vi "Configure Spot Frequency.vi"(0 "VISA resource name":refnum<visa-resource-name>, 1 "Spot Frequency Measurement Type (1: Signal Phase Noise)":i32(ring)=1 items=["Displayed Average Noise Level Floor", "Signal Phase Noise"], 2 "Video Resolution Bandwidth Ratio (1)":dbl=1.0, 3 "Average Count (0)":dbl, 4 "Averaging Method (0: Exponential)":i32(ring) items=["Exponential", "Repeat"], 5 "error in (no error)":errorcluster, 6 "Auto Phase Noise Optimization (T: Enable)":bool=TRUE, 7 "Spot Frequency Offset (10000 Hz)":dbl=10000.0 format="%^#_6g", 8 "Manual Phase Noise Optimization (45000 Hz)":dbl=45000.0 format="%^#_6g", 9 "Resolution Bandwidth (10%)":dbl=10.0, 11 "Sweep Time (0.005 s)":dbl=0.005) -> (14 "VISA resource name out":refnum<visa-resource-name>, 19 "error out":errorcluster)   [LabVIEW 2014, in "Agilent ESA PSA Series.lvlib"]
doc: "Configures the Spot Frequency measurement of the Phase Noise personality.\n\n<B>Note:</B>\n\nThis VI is only valid in Phase Noise personality. Use <B>Switch Personality</B> VI to switch to Phase Noise before calling this VI."
uses:
  Agilent ESA PSA Series.lvlib
panel:
  # "Only valid for PSA Models"
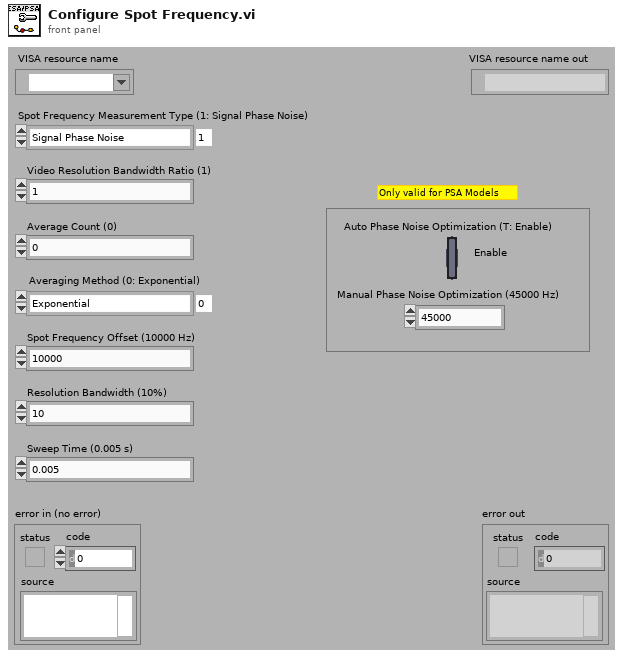
[diagram p1: front panel]
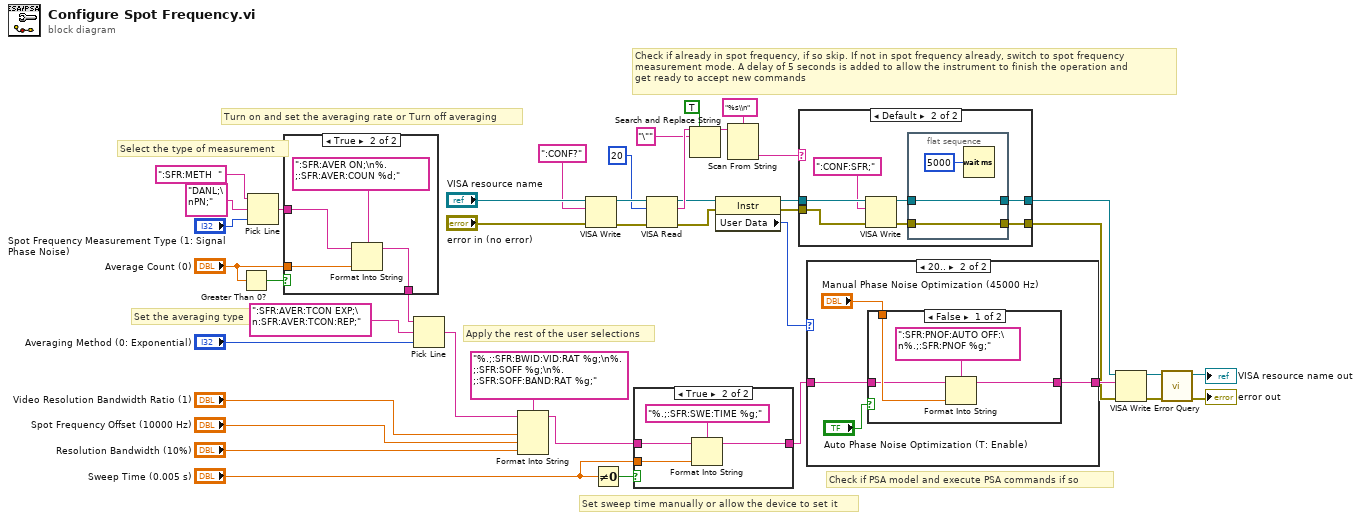
[diagram p0: block diagram]
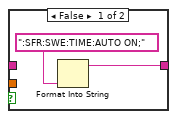
[diagram p3: hidden frame]
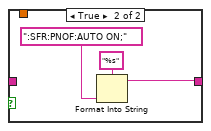
[diagram p5: hidden frame]
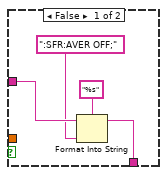
[diagram p6: hidden frame]
diagram:
  # "Check if already in spot frequency, if so skip. If not in spot frequency already, switch to spot frequency\nmeasurement mode. A delay of 5 seconds is added to allow the instrument to finish the operation and \nget ready to accept new commands"
  # "Set sweep time manually or allow the device to set it"
  # "Turn on and set the averaging rate or Turn off averaging"
  # "Set the averaging type"
  # "Apply the rest of the user selections"
  # "Select the type of measurement"
  # "Check if PSA model and execute PSA commands if so"
  n1 = Greater Than 0?(x="Average Count (0)") -> (x > 0?=w34:bool)
  n2 = Pick Line(string ("")=":SFR:METH  ", multi-line string="DANL;\nPN;", line index="Spot Frequency Measurement Type (1: Signal Phase Noise)") -> (output string=w35:string)
  n3 = case shown="True" w34 {
    tunnel: "Average Count (0)" -> [_ w50]
    tunnel: w35 -> [w46 w48]
    tunnel: [w45 w47] -> w30
    frame False {
      n4 = Format Into String(format string="%s", initial string=w46, ":SFR:AVER OFF;" ("input 1")) -> (resulting string=w45:string)  [unwired: 1 in, 1 out]
    }
    frame True {
      n5 = Format Into String(format string=":SFR:AVER ON;\n%.;:SFR:AVER:COUN %d;", initial string=w48, w50) -> (resulting string=w47:string)  [unwired: 1 in, 1 out]
    }
  }
  n6 = Pick Line(string ("")=w30, multi-line string=":SFR:AVER:TCON EXP;\n:SFR:AVER:TCON:REP;", line index="Averaging Method (0: Exponential)") -> (output string=w27:string)
  n7 = Format Into String(format string="%.;:SFR:BWID:VID:RAT %g;\n%.;:SFR:SOFF %g;\n%.;:SFR:SOFF:BAND:RAT %g;", initial string=w27, "Video Resolution Bandwidth Ratio (1)", "Spot Frequency Offset (10000 Hz)", "Resolution Bandwidth (10%)") -> (resulting string=w1:string)  [unwired: 1 in, 1 out]
  n8 = VISA Write(VISA resource name="VISA resource name", write buffer=":CONF?", error in (no error)="error in (no error)") -> (VISA resource name out=w12:refnum<visa-resource-name>, error out=w11:errorcluster)  [unwired: 1 out]
  n9 = Not Equal To 0?(x="Sweep Time (0.005 s)") -> (x != 0?=w25:bool)
  n10 = case shown="True" w25 {
    tunnel: "Sweep Time (0.005 s)" -> [_ w55]
    tunnel: [w51 w54] -> w23
    tunnel: w1 -> [_ w53]
    frame False {
      n11 = Format Into String(":SFR:SWE:TIME:AUTO ON;" ("format string")) -> (resulting string=w51:string)  [unwired: 3 in, 1 out]
    }
    frame True {
      n12 = Format Into String(format string="%.;:SFR:SWE:TIME %g;", initial string=w53, w55) -> (resulting string=w54:string)  [unwired: 1 in, 1 out]
    }
  }
  n13 = VISA Read(VISA resource name=w12, byte count=u32 20, error in (no error)=w11) -> (VISA resource name out=w8:refnum<visa-resource-name>, read buffer=w17:string, error out=w7:errorcluster)  [unwired: 1 out]
  n14 = Search and Replace String(replace all?=TRUE ("replace all? (F)"), input string=w17, search string="\"") -> (result string=w14:string)  [unwired: 5 in, 3 out]
  n15 = property class="Instr"(reference=w8, error in=w7) -> (reference out=w22:refnum<visa-resource-name>, error out=w21:errorcluster, "User Data"=w4:u32)
  n16 = Scan From String(format string="%s\\n", input string=w14) -> (output 1=w9:string)  [unwired: 3 in, 3 out]
  n17 = case shown="Default" w9 {
    tunnel: w22 -> [w58 w65]
    tunnel: w21 -> [w57 w64]
    tunnel: [w58 w61] -> w6
    tunnel: [w57 w60] -> w5
    frame "SFR", "SFRequency" {
    }
    frame Default {
      n18 = VISA Write(VISA resource name=w65, write buffer=":CONF:SFR;", error in (no error)=w64) -> (VISA resource name out=w63:refnum<visa-resource-name>, error out=w62:errorcluster)  [unwired: 1 out]
      n19 = flat-sequence {
        tunnel: w63 -> [w68]
        tunnel: w62 -> [w67]
        tunnel: [w68] -> w61
        tunnel: [w67] -> w60
        frame #0 {
          n20 = Wait (ms)(milliseconds to wait=u32 5000) -> ()  [unwired: 1 out]
        }
      }
    }
  }
  n21 = case shown="20.." w4 {
    tunnel: [w69 w71] -> w26
    tunnel: w23 -> [w69 w70]
    frame 0..19, Default {
      # "Not a PSA model, therefore skip PSA commands"
    }
    frame 20.. {
      n22 = case shown="False" "Auto Phase Noise Optimization (T: Enable)" {
        tunnel: [w77 w80] -> w71
        tunnel: "Manual Phase Noise Optimization (45000 Hz)" -> [w76 _]
        tunnel: w70 -> [w74 _]
        frame False {
          n23 = Format Into String(format string=":SFR:PNOF:AUTO OFF:\n%.;:SFR:PNOF %g;" ("input 1"), initial string=w74, w76) -> (resulting string=w77:string)  [unwired: 1 in, 1 out]
        }
        frame True {
          n24 = Format Into String(format string="%s", ":SFR:PNOF:AUTO ON;" ("format string")) -> (resulting string=w80:string)  [unwired: 2 in, 1 out]
        }
      }
    }
  }
  n25 = VISA Write(VISA resource name=w6, write buffer=w26, error in (no error)=w5) -> (VISA resource name out=w40:refnum<visa-resource-name>, error out=w39:errorcluster)  [unwired: 1 out]
  n26 = call "Error Query.vi"("error in (no error)"=w39, "VISA resource name"=w40) -> ("error out"=→"error out":errorcluster, "VISA resource name out"=→"VISA resource name out":refnum<visa-resource-name>)  [unwired: 6 in, 2 out]
